vi "escribeListaDePruebas.vi"(8 "error in (no error)":errorcluster, 11 "Calibrador in":refnum<class "Calibrador.lvclass">) -> (0 "error out":errorcluster, 3 "Calibrador out":refnum<class "Calibrador.lvclass">)   [LabVIEW 2019, in "Calibrador.lvclass"]
uses:
  Calibrador.lvclass
  C:/Users/ivan_/Documents/procal/Equipo/Equipo/Equipo.lvclass
  Calibrador.lvclass/Calibrador.ctl
  Base de Datos/Base de Datos.lvclass
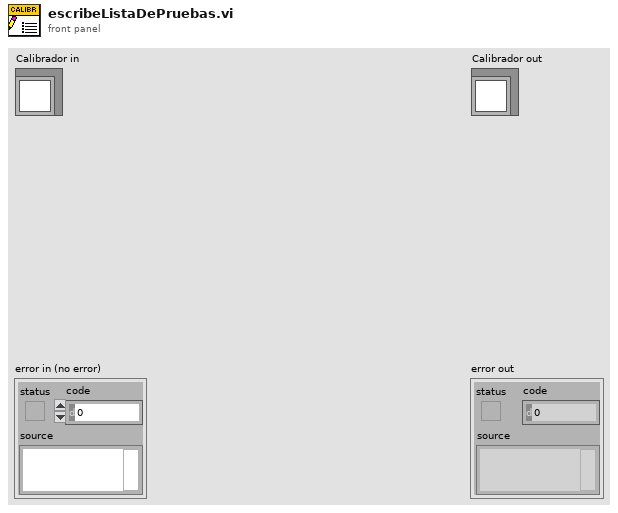
[diagram p1: front panel]
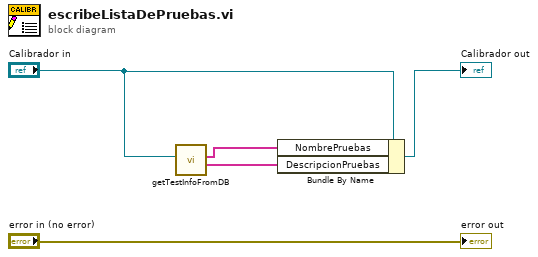
[diagram p0: block diagram]
diagram:
  n1 = call "getTestInfoFromDB.vi"("Equipo.lvclass"="Calibrador in") -> ("DescripcionPruebas"=w5:string[], "NombrePruebas"=w1:string[])  [unwired: 7 in, 2 out]
  n2 = Bundle By Name(cluster="Calibrador in", "NombrePruebas"=w1, "DescripcionPruebas"=w5) -> (→"Calibrador out":refnum<class "Calibrador.lvclass">)
  "error out" <- "error in (no error)"
